vi "Initialize.vi"(8 "error in (no error)":errorcluster, 9 "Fs (Hz)":dbl, 11 "Filter in":refnum<class "Filter.lvclass">) -> (0 "error out":errorcluster, 3 "Filter out":refnum<class "Filter.lvclass">)   [LabVIEW 2020, in "Filter.lvclass"]
uses:
  Filter.lvclass
  Filter.lvclass/Filter.ctl
  Shape.ctl
  392b410a-9c2b-41a3-9ff6-c08ec16ff704.vi
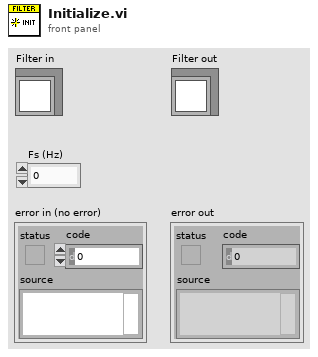
[diagram p1: front panel]
types:
  T1 = cluster{"IIR Filter Cluster":cluster{"filter structure":enum32{"IIR 2nd Order", "IIR 4th Order"}, "Reverse Coefficients":dbl[], "Forward Coefficients":dbl[]}, "Final Filter State":dbl[]}[]
  T2 = typedef "Filter.lvclass/Shape.ctl" = enum16{"OFF", "Lowpass", "Highpass", "Bandpass", "Bandstop"}
  T3 = typedef "Filter.lvclass/Units.ctl" = enum16{"Linear", "Octaves", "Min-Max"}
  T4 = typedef "Filter.lvclass/Class.ctl" = enum16{"Elliptic", "Butterworth", "Brickwall"}
  T5 = cluster{"IIR Filter Cluster":cluster{"filter structure":enum32{"IIR 2nd Order", "IIR 4th Order"}, "Reverse Coefficients":dbl[], "Forward Coefficients":dbl[]}, "Final Filter State":dbl[]}
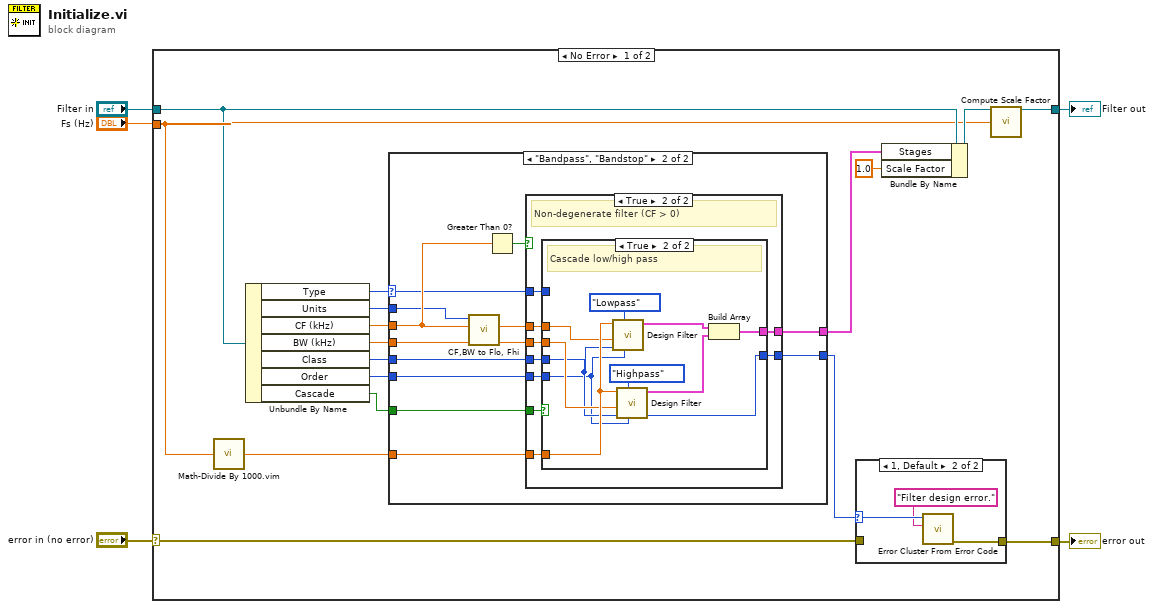
[diagram p0: block diagram]
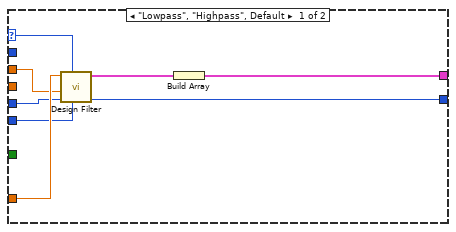
[diagram p2: hidden frame]
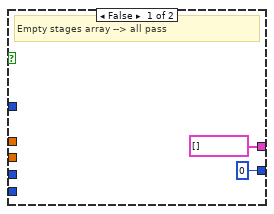
[diagram p3: hidden frame]
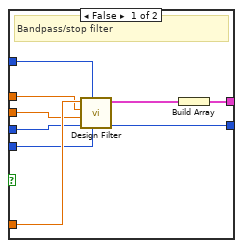
[diagram p4: hidden frame]
diagram:
  n1 = case shown="No Error" "error in (no error)" {
    selector: "error in (no error)" -> [w14 w80]
    tunnel: [w12 w80] -> w4
    tunnel: [w8 w79] -> w2
    tunnel: "Filter in" -> [w22 w79]
    tunnel: "Fs (Hz)" -> [w6 _]
    frame No Error {
      n2 = call "Math-Divide By 1000.vim"("X"=w6) -> ("1000X"=w7:dbl)
      n3 = Unbundle By Name(w22) -> ("Type"=w21:T2, "Units"=w20:T3, "CF (kHz)"=w19:dbl, "BW (kHz)"=w18:dbl, "Class"=w17:T4, "Order"=w16:i32, "Cascade"=w15:bool)
      n4 = case shown="\"Bandpass\", \"Bandstop\"" w21 {
        selector: w21 -> [w29 w35]
        tunnel: w19 -> [w23 w42]
        tunnel: w18 -> [_ w43]
        tunnel: w17 -> [w28 w39]
        tunnel: w16 -> [w27 w40]
        tunnel: [w25 w37] -> w11
        tunnel: w7 -> [w30 w41]
        tunnel: [w24 w38] -> w13
        tunnel: w15 -> [_ w36]
        tunnel: w20 -> [_ w34]
        frame "Lowpass", "Highpass", Default {
          n5 = call "Design Filter.vi"("order"=w27, "Type"=w29, "Class"=w28, "low cutoff freq: fl"=w23, "sampling freq: fs"=w30) -> ("error"=w24:i32, "IIR Filter"=w26:T5)  [unwired: 5 in]
          n6 = Build Array(w26) -> (w25:T1)
        }
        frame "Bandpass", "Bandstop" {
          n7 = call "CF,BW to Flo, Fhi.vi"("BW"=w43, "CF (kHz)"=w42, "BWUnits"=w34) -> ("Fmin"=w31:dbl, "Fmax"=w32:dbl)  [unwired: 7 in]
          n8 = Greater Than 0?(x=w42) -> (x > 0?=w33:bool)
          n9 = case shown="True" w33 {
            tunnel: w36 -> [_ w54]
            tunnel: w35 -> [_ w53]
            tunnel: w41 -> [_ w52]
            tunnel: w32 -> [_ w51]
            tunnel: w31 -> [_ w50]
            tunnel: w40 -> [_ w49]
            tunnel: w39 -> [_ w48]
            tunnel: [T1 [] w47] -> w37
            tunnel: [0 ("error") w46] -> w38
            frame False {
              # "Empty stages array --> all pass"
            }
            frame True {
              # "Non-degenerate filter (CF > 0)"
              n10 = case shown="True" w54 {
                tunnel: w53 -> [w55 _]
                tunnel: w52 -> [w63 w74]
                tunnel: w51 -> [w62 w73]
                tunnel: w50 -> [w61 w72]
                tunnel: w49 -> [w60 w66]
                tunnel: w48 -> [w59 w67]
                tunnel: [w58 w70] -> w47
                tunnel: [w56 w68] -> w46
                frame False {
                  # "Bandpass/stop filter"
                  n11 = call "Design Filter.vi"("order"=w60, "Type"=w55, "Class"=w59, "low cutoff freq: fl"=w61, "high cutoff freq: fh"=w62, "sampling freq: fs"=w63) -> ("error"=w56:i32, "IIR Filter"=w57:T5)  [unwired: 4 in]
                  n12 = Build Array(w57) -> (w58:T1)
                }
                frame True {
                  # "Cascade low/high pass"
                  n13 = call "Design Filter.vi"("order"=w66, "Type"=Shape."Lowpass", "Class"=w67, "low cutoff freq: fl"=w73, "sampling freq: fs"=w74) -> ("IIR Filter"=w71:T5)  [unwired: 5 in, 1 out]
                  n14 = call "Design Filter.vi"("order"=w66, "Type"=Shape."Highpass", "Class"=w67, "low cutoff freq: fl"=w72, "sampling freq: fs"=w74) -> ("error"=w68:i32, "IIR Filter"=w69:T5)  [unwired: 5 in]
                  n15 = Build Array(w71, w69) -> (w70:T1)
                }
              }
            }
          }
        }
      }
      n16 = case shown="1, Default" w13 {
        selector: w13 -> [_ w78]
        tunnel: [w75 w77] -> w12
        tunnel: w14 -> [w75 _]
        frame 0 {
        }
        frame 1, Default {
          n17 = call <vilib>:"Error Cluster From Error Code.vi"("error message (\"\")"="Filter design error." ("error message (\"\")"), "error code (0)"=w78) -> ("error out"=w77:errorcluster)  [unwired: 7 in]
        }
      }
      n18 = Bundle By Name(cluster=w22, "Stages"=w11, "Scale Factor"=1.0) -> (w9:refnum<class "Filter.lvclass">)
      n19 = call "Compute Scale Factor.vi"("Filter"=w9, "Sampling Rate (Hz)"=w6) -> ("Filter out"=w8:refnum<class "Filter.lvclass">)  [unwired: 12 in, 1 out]
    }
    frame Error {
    }
  }
  "error out" <- w4
  "Filter out" <- w2
